vi "ICSETTINGS_write.vi"(8 "error in (no error)":errorcluster, 9 "ICSETINGS":T2, 10 "MAINHARDWAREHDR":T1, 11 "refnum in":refnum<file>) -> (0 "error out":errorcluster, 3 "refnum out":refnum<file>)   [LabVIEW 2012]
uses:
  TTTR_data_headers/ICSETTINGS.ctl
  TTTR_data_headers/MAINHARDWAREHDR.ctl
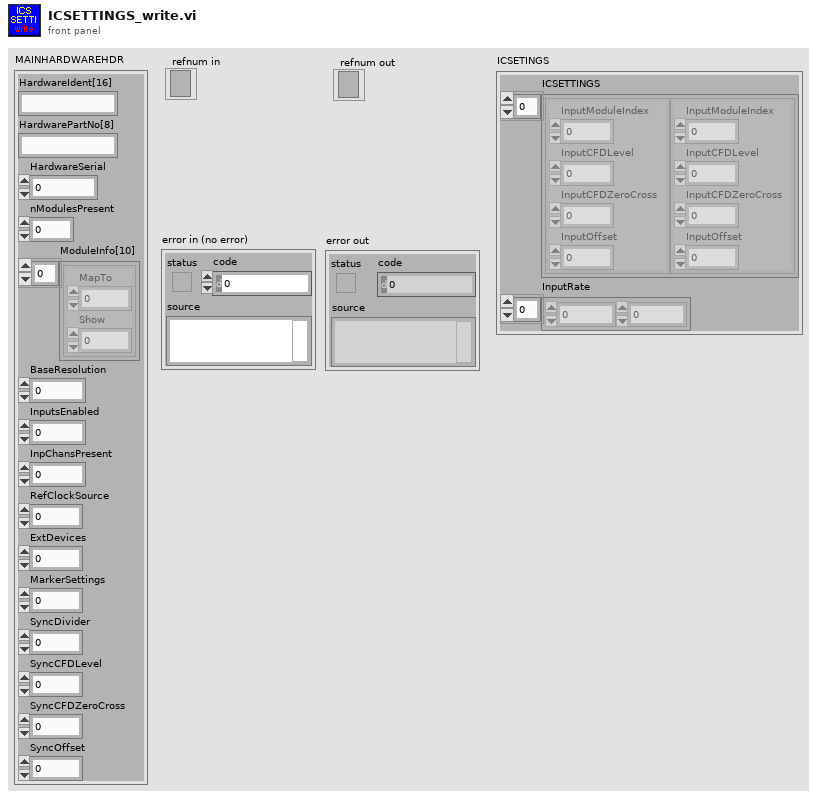
[diagram p1: front panel]
types:
  T1 = typedef "MAINHARDWAREHDR.ctl" = cluster{"HardwareIdent[16]":string, "HardwarePartNo[8]":string, "HardwareSerial":i32, "nModulesPresent":i32, "ModuleInfo[10]":cluster{"MapTo":i32, "Show":i32}[], "BaseResolution":dbl, "InputsEnabled":u64, "InpChansPresent":i32, "RefClockSource":i32, "ExtDevices":i32, "MarkerSettings":i32, "SyncDivider":i32, "SyncCFDLevel":i32, "SyncCFDZeroCross":i32, "SyncOffset":i32}
  T2 = typedef "ICSETTINGS.ctl" = cluster{"ICSETTINGS":cluster{"InputModuleIndex":i32, "InputCFDLevel":i32, "InputCFDZeroCross":i32, "InputOffset":i32}[], "InputRate":i32[]}
  T3 = enum16{"big-endian, network order", "native, host order", "little-endian"}
  T4 = cluster{"InputModuleIndex":i32, "InputCFDLevel":i32, "InputCFDZeroCross":i32, "InputOffset":i32}[]
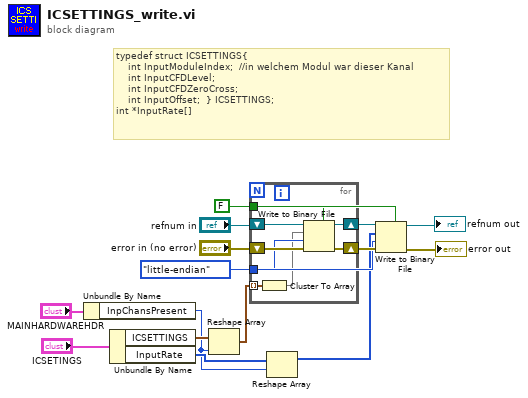
[diagram p0: block diagram]
diagram:
  w1 = FALSE ("prepend array or string size? (T)")
  w13 = T3."little-endian" ("byte order (0:big-endian, network order)")
  # "typedef struct ICSETTINGS{ \n\t\t\t\tint InputModuleIndex;  //in welchem Modul war dieser Kanal\n\t\t\t\tint InputCFDLevel;\n\t\t\t\tint InputCFDZeroCross; \n\t\t\t\tint InputOffset;\t\t} ICSETTINGS; \nint *InputRate[]"
  n1 = Unbundle By Name("MAINHARDWAREHDR") -> ("InpChansPresent"=w3:i32)
  n2 = Unbundle By Name("ICSETINGS") -> ("ICSETTINGS"=w5:T4, "InputRate"=w6:i32[])
  n3 = Reshape Array(w5, w3) -> (w2:T4)
  n4 = for {
    shift-right: [w20] -> w15
    shift-left: "error in (no error)" -> [w23]
    shift-right: [w21] -> w14
    shift-left: "refnum in" -> [w22]
    tunnel: w13 -> [w19]
    tunnel: w2 -> [w17] mode=indexing
    tunnel: w1 -> [w18]
    n5 = Cluster To Array(cluster=w17) -> (array=w16:i32[])
    n6 = Write to Binary File(file (use dialog)=w22, data=w16, error in=w23, 5:w18, 9:w19) -> (refnum out=w21:refnum<file>, error out=w20:errorcluster)  [unwired: 1 in, 1 out]
  }
  n7 = Reshape Array(w6, w3) -> (w4:i32[])
  n8 = Write to Binary File(file (use dialog)=w14, data=w4, error in=w15, 5:w1, 9:w13) -> (refnum out=→"refnum out":refnum<file>, error out=→"error out":errorcluster)  [unwired: 1 in, 1 out]
